vi "Add Start and Stop Channels.vi"(8 "error in":errorcluster, 11 "terminal":T1 format="%.0x") -> (0 "error out":errorcluster, 1 "stop command channel":T1 format="%.0x", 2 "start command channel":T1 format="%.0x", 3 "terminal out":T1 format="%.0x")   [LabVIEW 2020, in "AIM MIL-STD-1553 Scripting.lvlib"]
doc: "Adds two command channels to specified terminal, named \"Start\" and \"Stop\", and returns references to those command channels."
uses:
  AIM MIL-STD-1553 Scripting.lvlib
  <vilib>/NI VeriStand/Custom Device API/Custom Device Item Ref.ctl
  Constants.vi
  <vilib>/NI VeriStand/Custom Device API/Custom Device API.lvlib
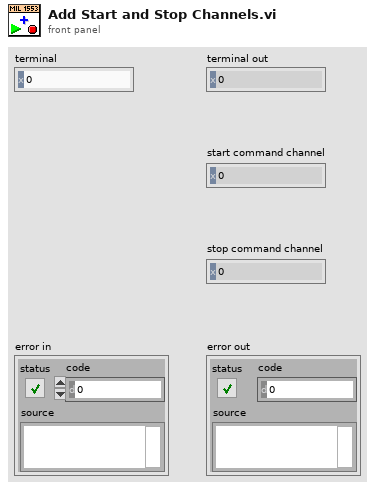
[diagram p1: front panel]
types:
  T1 = typedef "Custom Device API.lvlib/Custom Device Item Ref.ctl" = u64
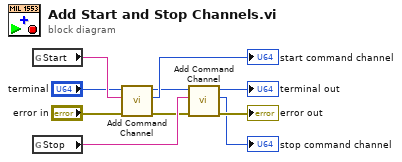
[diagram p0: block diagram]
diagram:
  n1 = global read "Constants.vi" "Start"() -> (w8:string)
  n2 = global read "Constants.vi" "Stop"() -> (w9:string)
  n3 = call "Add Command Channel.vi"("error in"="error in", "name"=w8, "terminal"="terminal") -> ("error out"=w7:errorcluster, "command channel"=→"start command channel":T1, "terminal out"=w3:T1)  [unwired: 6 in]
  n4 = call "Add Command Channel.vi"("error in"=w7, "name"=w9, "terminal"=w3) -> ("error out"=→"error out":errorcluster, "command channel"=→"stop command channel":T1, "terminal out"=→"terminal out":T1)  [unwired: 6 in]
